vi "svx_Waterfall Add Cursor.vi"(0 "cursors":T1[](array[typedef]), 1 "cursor points":cluster{"X":dbl, "Y":dbl, "Z":dbl}[](array[cluster]), 5 "error in (no error)":errorcluster) -> (14 "appended cursors":T1[](array[typedef]), 15 "duplicate cursor points":cluster{"X":dbl, "Y":dbl, "Z":dbl}[](array[cluster]), 17 "cursor index":i32, 19 "error out":errorcluster)   [LabVIEW 2017]
uses:
  <vilib>/addons/_NISVFA/_Shared subVIs/Controls/svc_Cluster of Array of Cluster of XYZ.ctl
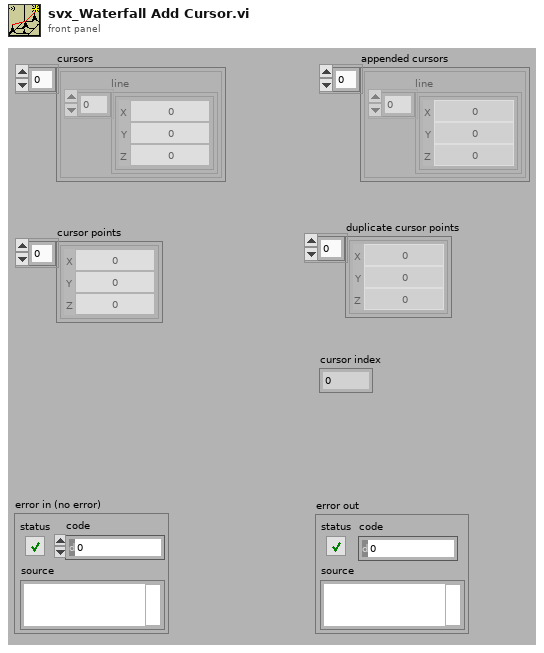
[diagram p1: front panel]
types:
  T1 = typedef "svc_Cluster of Array of Cluster of XYZ.ctl" = cluster{"line":cluster{"X":dbl, "Y":dbl, "Z":dbl}[]}
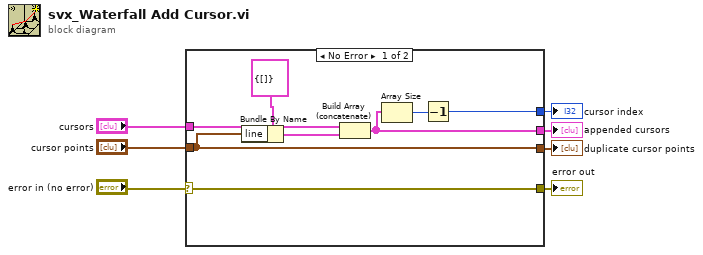
[diagram p0: block diagram]
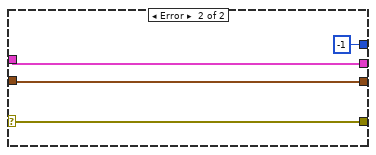
[diagram p2: hidden frame]
diagram:
  n1 = case shown="No Error" "error in (no error)" {
    selector: "error in (no error)" -> [w8 w17]
    tunnel: [w8 w17] -> w5
    tunnel: "cursors" -> [w14 w18]
    tunnel: [w12 w18] -> w3
    tunnel: [w10 -1] -> w1
    tunnel: "cursor points" -> [w9 w16]
    tunnel: [w9 w16] -> w4
    frame No Error {
      n2 = Bundle By Name(cluster=T1 {"line"=[]}, "line"=w9) -> (w13:T1)
      n3 = Build Array (concatenate)(w14, w13) -> (w12:T1[])
      n4 = Array Size(array=w12) -> (size(s)=w11:i32)
      n5 = Decrement(x=w11) -> (x-1=w10:i32)
    }
    frame Error {
    }
  }
  "error out" <- w5
  "duplicate cursor points" <- w4
  "appended cursors" <- w3
  "cursor index" <- w1
